vi "Temp Viewer.vi"() -> ()   [LabVIEW 2017, in "DSF Core.lvlib"]
uses:
  DSF Core.lvlib
  Typedefs/DSF Engine Framework Configuration.ctl
  Typedefs/DSF Engine Plugin Configuration.ctl
  Typedefs/DSF Timing Info.ctl
  Typedefs/DSF Engine Plugin Thread Configuration.ctl
  Typedefs/DSF Settings Info.ctl
  Typedefs/DSF Engine Transfer Group Configuration.ctl
  Typedefs/DSF Direction.ctl
  Typedefs/DSF Engine Transfer Configuration.ctl
  Typedefs/DSF Byte Order.ctl
  Typedefs/DSF Engine Channel Configuration.ctl
  Typedefs/DSF Data Type.ctl
  Typedefs/DSF Timeout Behavior.ctl
  Classes/Thread/Data Server/DSF Buffer Subset Descriptor.ctl
  Typedefs/DSF Buffer Type.ctl
panel:
  out "framework configuration":T1
  in  "stop":bool
  out "data":string
  out "timed out?":bool
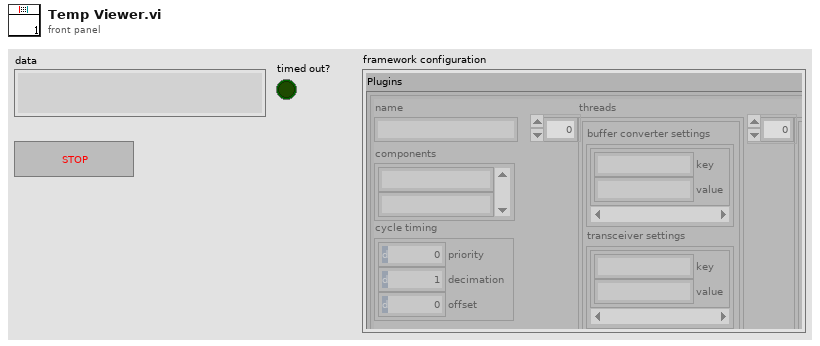
[diagram p1: front panel]
types:
  T1 = typedef "DSF Core.lvlib/DSF Engine Framework Configuration.ctl" = cluster{"Plugins":T2[]}
  T2 = typedef "DSF Core.lvlib/DSF Engine Plugin Configuration.ctl" = cluster{"name":string, "components":string[], "cycle timing":T3, "threads":T4[], "Transfer Groups":T6[], "settings":T5}
  T3 = typedef "DSF Core.lvlib/DSF Timing Info.ctl" = cluster{"priority":u64, "decimation":u64, "offset":u64}
  T4 = typedef "DSF Core.lvlib/DSF Engine Plugin Thread Configuration.ctl" = cluster{"buffer converter settings":T5, "transceiver settings":T5, "custom settings":T5, "processor":i32, "priority offset":i16}
  T5 = typedef "DSF Core.lvlib/DSF Settings Info.ctl" = cluster{"key":string, "value":string}[]
  T6 = typedef "DSF Core.lvlib/DSF Engine Transfer Group Configuration.ctl" = cluster{"name":string, "direction":T7, "cycle timing":T3, "thread index":i32, "settings":T5, "Transfers":T8[], "timeout behavior":T12}
  T7 = typedef "DSF Core.lvlib/DSF Direction.ctl" = enum8{"Tx", "Rx"}
  T8 = typedef "DSF Core.lvlib/DSF Engine Transfer Configuration.ctl" = cluster{"name":string, "byte order":T9, "settings":T5, "channels":T10[]}
  T9 = typedef "DSF Core.lvlib/DSF Byte Order.ctl" = enum8{"big-endian", "little-endian"}
  T10 = typedef "DSF Core.lvlib/DSF Engine Channel Configuration.ctl" = cluster{"string offset":u64, "string data type":T11, "engine data type":T11, "name":string, "settings":T5, "units":string}
  T11 = typedef "DSF Core.lvlib/DSF Data Type.ctl" = enum8{"Bool", "SGL", "DBL", "I8", "I16", "I32", "I64", "U8", "U16", "U32", "U64"}
  T12 = typedef "DSF Core.lvlib/DSF Timeout Behavior.ctl" = enum8{"Increment Late Count", "Throw Error"}
  T13 = typedef "DSF Core.lvlib/DSF Buffer Subset Descriptor.ctl" = cluster{"buffer type":T14, "plugin id":i32, "group id":i32, "transfer id":i32, "offset":u64, "length":i64}
  T14 = typedef "DSF Core.lvlib/DSF Buffer Type.ctl" = enum16{"Engine", "String"}
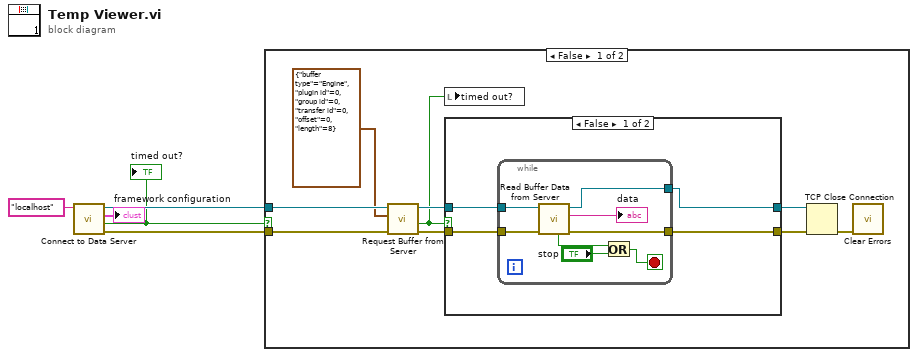
[diagram p0: block diagram]
diagram:
  n1 = call "Connect to Data Server.vi"("server address"="localhost") -> ("error out"=w2:errorcluster, "timed out?"=w3:bool, "framework configuration"=→"framework configuration":T1, "server ID"=w4:refnum<k5>)  [unwired: 7 in]
  "timed out?" <- w3
  n2 = case shown="False" w3 {
    tunnel: w4 -> [w13 _]
    tunnel: w2 -> [w14 _]
    frame False {
      n3 = call "Request Buffer from Server.vi"("error in (no error)"=w14, "buffer descriptor"=T13 {"buffer type"=enum."Engine", "plugin id"=0, "group id"=0, "transfer id"=0, "offset"=0, "length"=8}, "server ID in"=w13) -> ("error out"=w10:errorcluster, "timed out?"=w9:bool, "server ID out"=w11:refnum<k5>)  [unwired: 6 in]
      n4 = local write "timed out?"(w9) -> ()
      n5 = case shown="False" w9 {
        tunnel: w11 -> [w18 w28]
        tunnel: w10 -> [w17 w27]
        tunnel: [w16 w27] -> w8
        tunnel: [w15 w28] -> w7
        frame False {
          n6 = while {
            tunnel: w18 -> [w26]
            tunnel: w17 -> [w25]
            tunnel: [w21] -> w15
            tunnel: [w20] -> w16
            stop <- w22 stop-if-true
            n7 = call "Read Buffer Data from Server.vi"("error in (no error)"=w25, "server ID in"=w26) -> ("error out"=w20:errorcluster, "buffer data"=→"data":string, "server ID out"=w21:refnum<k5>, "timed out?"=w19:bool)  [unwired: 5 in, 1 out]
            n8 = Or(x=w19, y="stop") -> (x .or. y?=w22:bool)
          }
        }
        frame True {
        }
      }
      n9 = TCP Close Connection(connection ID=w7, error in (no error)=w8) -> (error out=w6:errorcluster)  [unwired: 1 in, 1 out]
      n10 = call <vilib>:"Clear Errors.vi"("error in (no error)"=w6) -> ()  [unwired: 5 in, 2 out]
    }
    frame True {
    }
  }
